vi "mate std to unknown simple.vi"(8 "error in":errorcluster, 11 "cycle results cluster result":T1 {"cycle results dbl" format="%#_6e"}) -> (0 "error out":errorcluster, 3 "output cluster":T1 {"cycle results dbl" format="%#_11f"})   [LabVIEW 2016]
uses:
  controls/cycle results control.ctl
panel:
  out "Array":dbl[][](array[numeric])
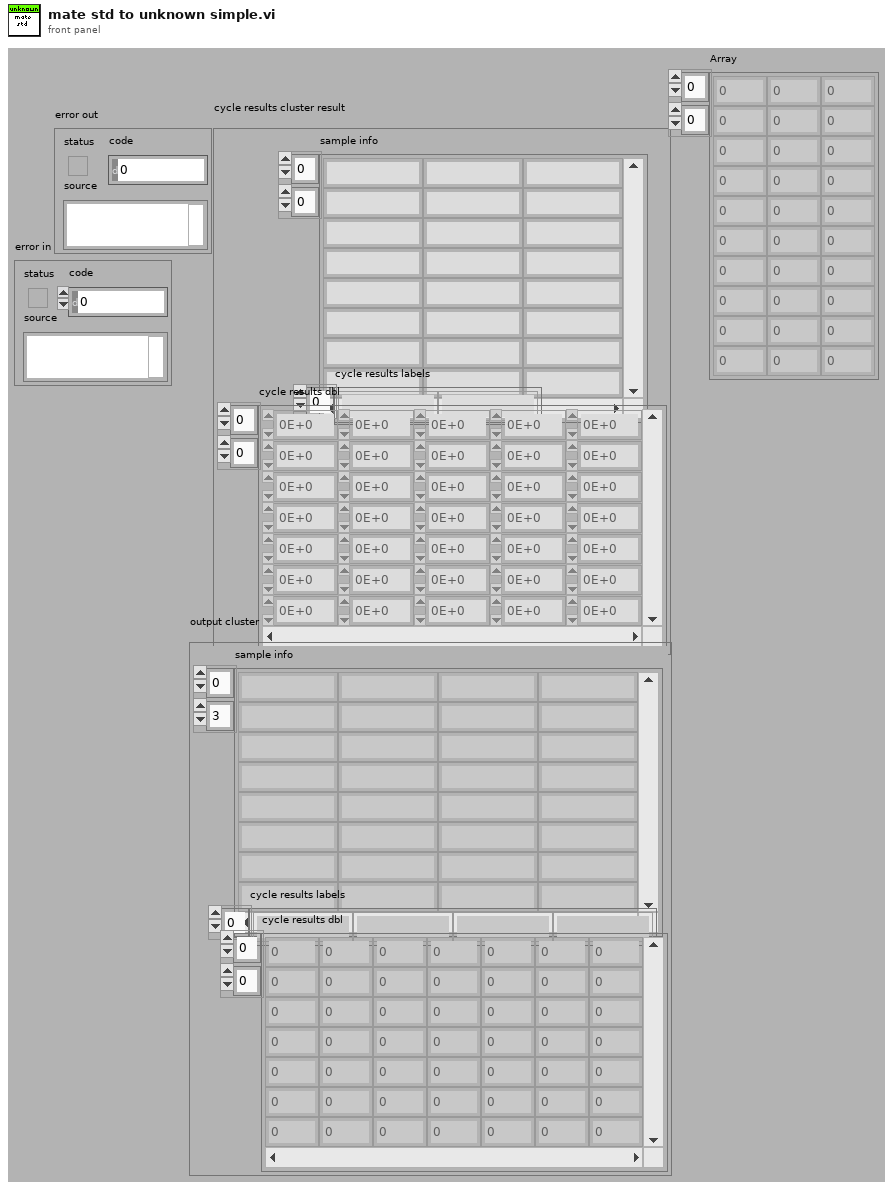
[diagram p1: front panel]
types:
  T1 = typedef "cycle results control.ctl" = cluster{"sample info":string[][], "cycle results labels":string[], "cycle results dbl":dbl[][]}
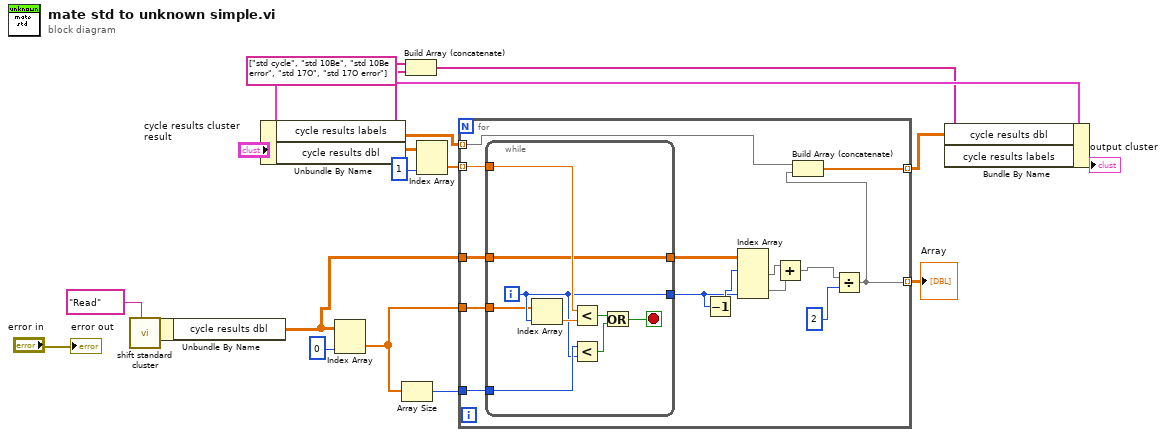
[diagram p0: block diagram]
diagram:
  n1 = call "shift standard cluster.vi"("read write shift"="Read") -> ("cycle results cluster out"=w15:T1)  [unwired: 9 in, 1 out]
  n2 = Unbundle By Name(w15) -> ("cycle results dbl"=w10:dbl[][])
  n3 = Unbundle By Name("cycle results cluster result") -> ("cycle results labels"=w5:string[], "cycle results dbl"=w9:dbl[][])
  n4 = Index Array(array=w10, index (col)=0 ("disabled index (col)")) -> (element=w11:dbl[])  [unwired: 1 in]
  n5 = Array Size(array=w11) -> (size(s)=w12:i32)
  n6 = Build Array (concatenate)(w5, string[] ["std cycle", "std 10Be", "std 10Be error", "std 17O", "std 17O error"] ("element")) -> (w3:string[])
  n7 = Index Array(array=w9, index (col)=1 ("disabled index (col)")) -> (element=w13:dbl[])  [unwired: 1 in]
  n8 = for {
    tunnel: w11 -> [w31]
    tunnel: w13 -> [w30] mode=indexing
    tunnel: w12 -> [w29]
    tunnel: w10 -> [w24]
    tunnel: w9 -> [w21] mode=indexing
    tunnel: [w20] -> w7 mode=indexing
    tunnel: [w18] -> w1 mode=indexing
    n9 = while {
      tunnel: w31 -> [w33]
      tunnel: w30 -> [w39]
      tunnel: w29 -> [w40]
      tunnel: [w34] -> w19
      tunnel: [w32] -> w28
      tunnel: w24 -> [w32]
      i -> [w34]
      stop <- w35 stop-if-true
      n10 = Index Array(array=w33, index=w34) -> (element=w38:dbl)
      n11 = Less?(x=w39, y=w38) -> (x < y?=w36:bool)
      n12 = Less?(x=w40, y=w34) -> (x < y?=w37:bool)
      n13 = Or(x=w36, y=w37) -> (x .or. y?=w35:bool)
    }
    n14 = Decrement(x=w19) -> (x-1=w27:i32)
    n15 = Index Array(array=w28, index (row) #1=w27, index (row) #2=w19) -> (element #1=w25:dbl[], element #2=w26:dbl[])  [unwired: 2 in]
    n16 = Add(x=w25, y=w26) -> (x+y=w23:dbl[])
    n17 = Divide(x=w23, y=2 ("String")) -> (x/y=w18:dbl[])
    n18 = Build Array (concatenate)(w21, w18) -> (w20:dbl[])
  }
  "Array" <- w1
  n19 = Bundle By Name(cluster="cycle results cluster result", "cycle results dbl"=w7, "cycle results labels"=w3) -> (→"output cluster":T1)
  "error out" <- "error in"
